vi "Test Event Handling.vi"() -> ()   [LabVIEW 2021]
uses:
  <vilib>/event_ctls.llb/usereventprio.ctl
panel:
  out "value 2":bool
  out "Numeric 3":i32
  out "Numeric 2":i32
  out "Numeric":i32
  in  "stop 2":bool
  in  "Value":bool
  out "value":bool
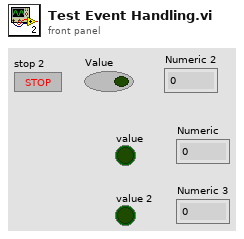
[diagram p1: front panel]
types:
  T1 = typedef "usereventprio.ctl" = enum32{"high priority", "normal priority"}
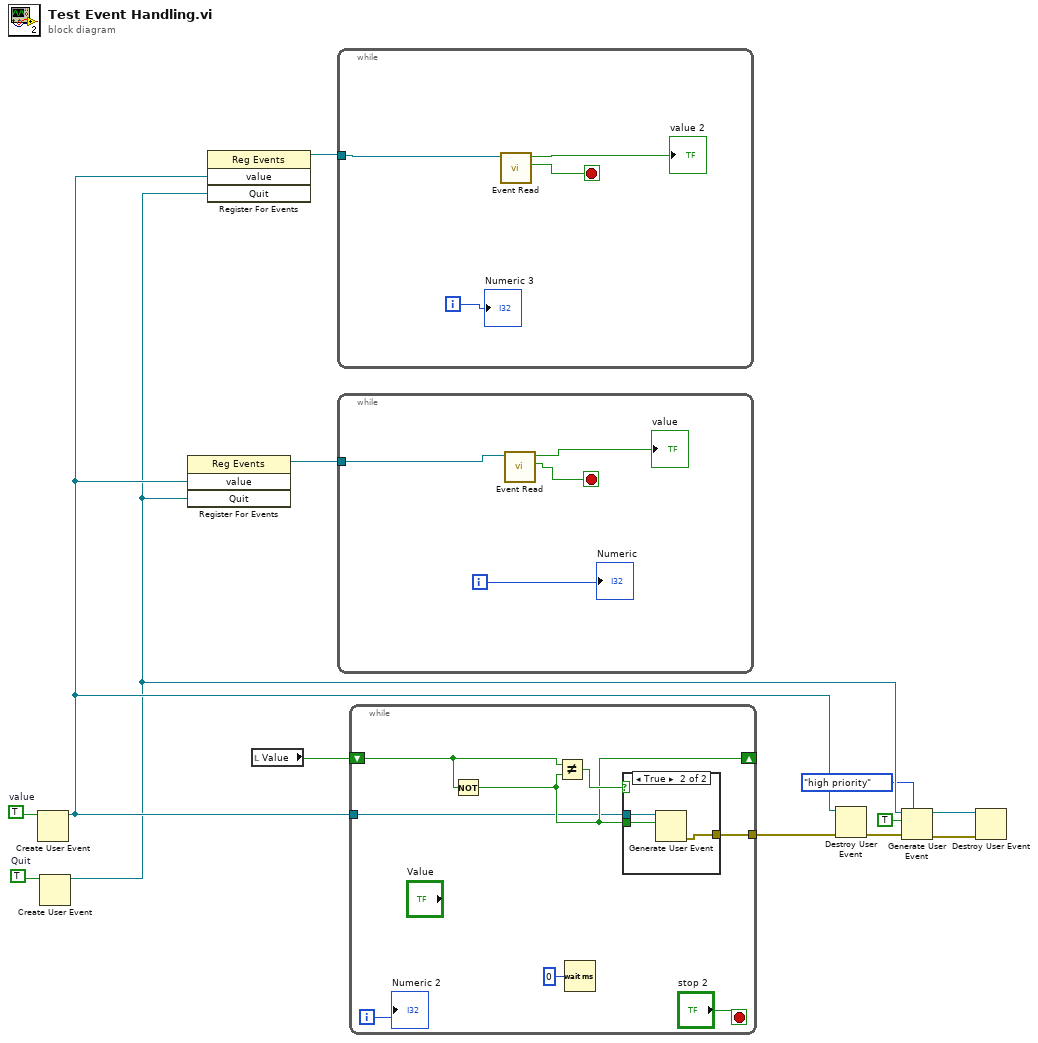
[diagram p0: block diagram]
diagram:
  w11 = TRUE  # Quit
  w13 = TRUE  # value
  n1 = Create User Event(user event datatype=w13) -> (user event=w3:refnum<user-event>)  [unwired: 1 in, 1 out]
  n2 = Create User Event(user event datatype=w11) -> (user event=w2:refnum<user-event>)  [unwired: 1 in, 1 out]
  n3 = register-events(w3, w2) -> (reference out=w5:refnum<event-registration>)  [unwired: 2 in, 1 out]
  n4 = register-events(w3, w2) -> (reference out=w4:refnum<event-registration>)  [unwired: 2 in, 1 out]
  n5 = local read "Value"() -> (w6:bool)
  n6 = while {
    tunnel: w4 -> [w17]
    i -> [w16]
    stop <- w14 stop-if-true
    n7 = call "Event Read.vi"("Event Registration Refnum in"=w17) -> ("Quit"=w14:bool, "value"=→"value 2":bool)  [unwired: 9 in]
    "Numeric 3" <- w16
  }
  n8 = while {
    tunnel: w5 -> [w18]
    i -> [w21]
    stop <- w19 stop-if-true
    n9 = call "Event Read.vi"("Event Registration Refnum in"=w18) -> ("Quit"=w19:bool, "value"=→"value":bool)  [unwired: 9 in]
    "Numeric" <- w21
  }
  n10 = while {
    tunnel: w3 -> [w22]
    tunnel: [w28] -> w12
    shift-right: [w23] -> _
    shift-left: w6 -> [w24]
    i -> [w26]
    stop <- "stop 2" stop-if-true
    n11 = Not(x=w24) -> (.not. x?=w23:bool)
    n12 = Not Equal?(x=w24, y=w23) -> (x != y?=w25:bool)
    n13 = Wait (ms)(milliseconds to wait=u32 0) -> ()  [unwired: 1 out]
    n14 = case shown="True" w25 {
      tunnel: w22 -> [_ w32]
      tunnel: [_ w31] -> w28
      tunnel: w23 -> [_ w30]
      frame False {
      }
      frame True {
        n15 = Generate User Event(user event=w32, event data cluster=w30) -> (error out=w31:errorcluster)  [unwired: 2 in, 1 out]
      }
    }
    "Numeric 2" <- w26
  }
  n16 = Destroy User Event(user event=w3, error in=w12) -> (error out=w10:errorcluster)
  n17 = Generate User Event(priority (normal)=usereventprio."high priority", user event=w2, event data cluster=TRUE ("event data"), error in=w10) -> (user event out=w7:refnum<user-event>, error out=w8:errorcluster)
  n18 = Destroy User Event(user event=w7, error in=w8) -> ()  [unwired: 1 out]
